vi "Initialize FPGA.vi"(8 "error in (no error)":errorcluster) -> (0 "error out":errorcluster, 3 "FPGA VI Reference":T1)   [LabVIEW 2014]
uses:
  controls/FPGA VI Reference.ctl
  <vilib>/FPGAPlugInAG/cRIO-9114/niLvFpga_Open_cRIO-9114.vi
  <vilib>/rvi/interface/common/dynamic/niFpgaDynamicAddResources.vi
  <vilib>/FPGAPlugInAG/Dynamic/niLvFpga_Reset_Dynamic.vi
  <vilib>/rvi/interface/nirviOpenFPGA/nirviOpenFPGA.xnode
  FPGA Bitfiles/FreiaInterlock_FPGATarget_FPGAMain_d9emsL9JL5U.lvbitx
  <vilib>/rvi/interface/nirviMethod/nirviMethod.xnode
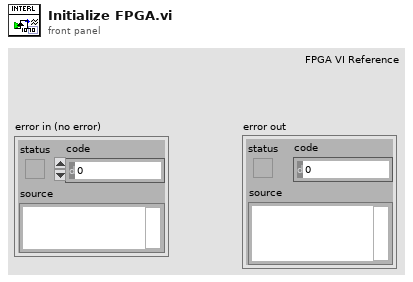
[diagram p1: front panel]
types:
  T1 = typedef "FPGA VI Reference.ctl" = refnum<k20>
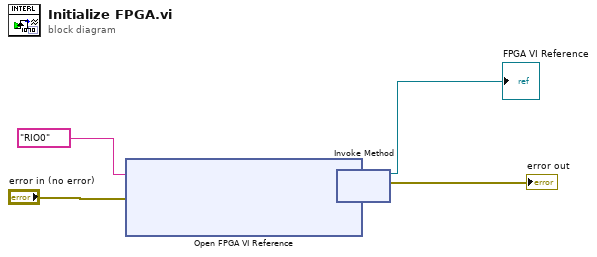
[diagram p0: block diagram]
diagram:
  n1 = xnode "Open FPGA VI Reference"("error in"="error in (no error)", "resource name"=tag "RIO0") -> ("FPGA VI Reference Out"=w5:refnum<k20>, "error out"=w4:errorcluster)
  n2 = xnode "Invoke Method"("FPGA VI Reference In"=w5, "error in"=w4) -> ("FPGA VI Reference Out"=→"FPGA VI Reference":refnum<k20>, "error out"=→"error out":errorcluster)
